vi "Send Close Event.vi"(8 "error in (no error)":errorcluster, 11 "QMenu Class in":refnum<class "QMenu Class.lvclass">) -> (0 "error out":errorcluster, 2 "Confirm":bool, 3 "QMenu Class out":refnum<class "QMenu Class.lvclass">)   [LabVIEW 2020, in "QTab.lvlib" / "QMenu Class.lvclass"]
uses:
  QMenu Class.lvclass
  QMenu Class.lvclass/QMenu Class.ctl
  Close Event Data.ctl
  Read Close Timeout.vi
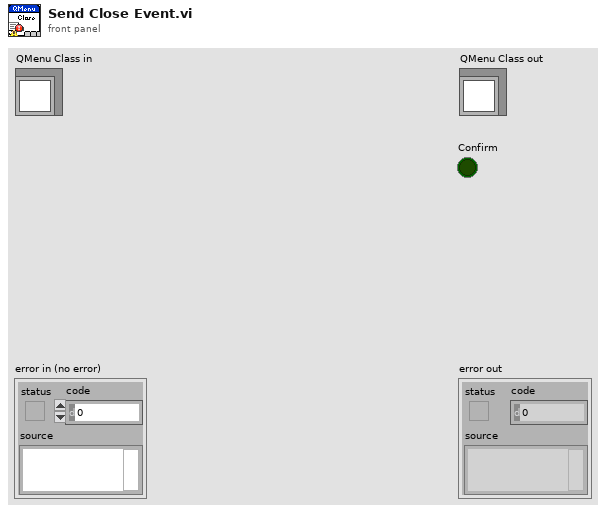
[diagram p1: front panel]
types:
  T1 = typedef "QTab.lvlib/QMenu Class.lvclass/Close Event Data.ctl" = cluster{"Index":i32, "Label":string, "Confirm Notifier":refnum<notifier>}
  T2 = typedef "QTab.lvlib/QMenu Class.lvclass/Button Attribute.ctl" = cluster{"Label":string, "Button Text":string, "Closable":bool, "Draggable":bool}
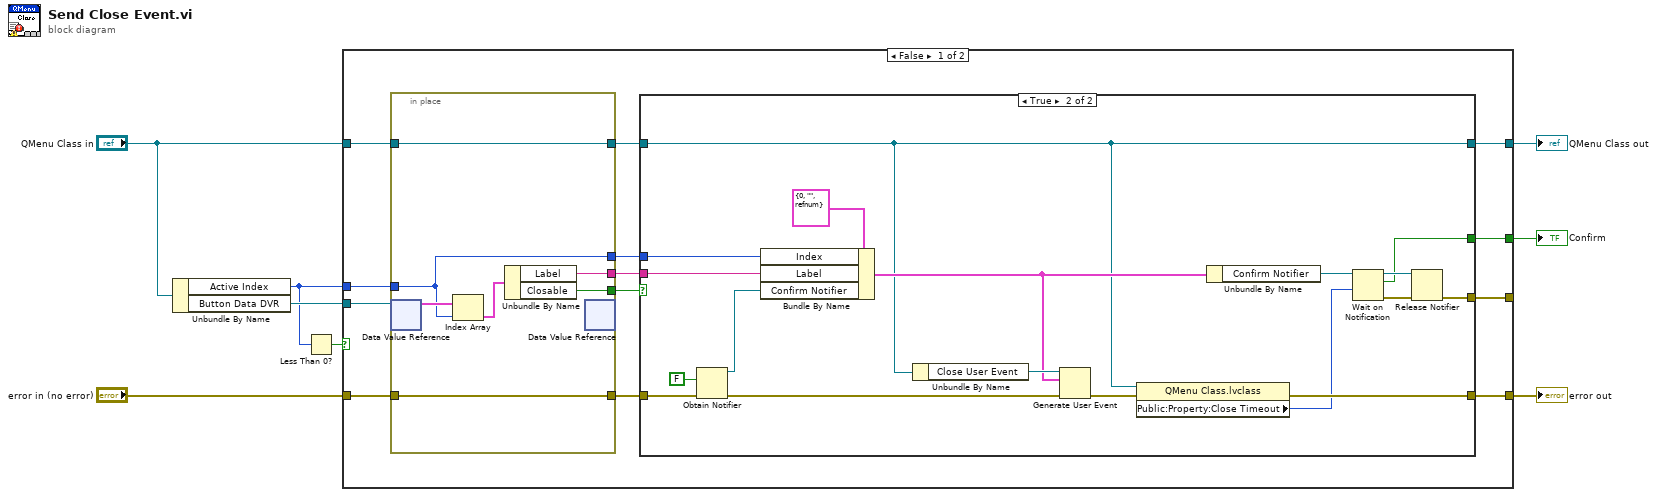
[diagram p0: block diagram]
diagram:
  n1 = Unbundle By Name("QMenu Class in") -> ("Active Index"=w3:i32, "Button Data DVR"=w7:refnum<data-value>)
  n2 = Less Than 0?(x=w3) -> (x < 0?=w2:bool)
  n3 = case shown="False" w2 {
    tunnel: [w12 w49] -> w8
    tunnel: w7 -> [w21 _]
    tunnel: "error in (no error)" -> [w20 w49]
    tunnel: "QMenu Class in" -> [w19 w50]
    tunnel: [w9 w50] -> w4
    tunnel: w3 -> [w17 _]
    tunnel: [w13 _] -> _
    tunnel: [w11 _] -> w1
    frame False {
      n4 = in-place {
        in-place-border: w17 -> [w44]
        in-place-border: w20 -> [w45]
        in-place-border: w19 -> [w48]
        in-place-border: [w48] -> w18
        in-place-border: [w45] -> w16
        in-place-border: [w44] -> w15
        in-place-border: [w43] -> w14
        in-place-border: [w42] -> w10
        n5 = in-place-dvr #1(w21) -> (w47:T2[])  [unwired: 1 out]
        n6 = Index Array(array=w47, index=w44) -> (element=w46:T2)
        n7 = Unbundle By Name(w46) -> ("Label"=w43:string, "Closable"=w42:bool)
        n8 = in-place-dvr #1() -> ()  [unwired: 1 in, 2 out]
      }
      n9 = case shown="True" w10 {
        tunnel: w18 -> [w22 w26]
        tunnel: w16 -> [w23 w40]
        tunnel: w15 -> [_ w36]
        tunnel: w14 -> [_ w35]
        tunnel: [_ w29] -> w13
        tunnel: [w23 w25] -> w12
        tunnel: [_ w28] -> w11
        tunnel: [w22 w26] -> w9
        frame False {
        }
        frame True {
          n10 = Obtain Notifier(notification data type=FALSE, error in (no error)=w40) -> (notifier out=w37:refnum<notifier>, error out=w34:errorcluster)  [unwired: 2 in, 1 out]
          n11 = Bundle By Name(cluster=T1 {"Index"=0, "Label"="", "Confirm Notifier"=refnum} ("Close Event Data"), "Index"=w36, "Label"=w35, "Confirm Notifier"=w37) -> (w33:T1)
          n12 = Unbundle By Name(w26) -> ("Close User Event"=w41:refnum<user-event>)
          n13 = Generate User Event(user event=w41, event data cluster=w33, error in=w34) -> (error out=w27:errorcluster)  [unwired: 1 in, 1 out]
          n14 = property class="QMenu Class.lvclass"(reference=w26, error in=w27) -> (error out=w25:errorcluster, "Public:Property:Close Timeout"=w24:i32)  [unwired: 1 out]
          n15 = Unbundle By Name(w33) -> ("Confirm Notifier"=w32:refnum<notifier>)
          n16 = Wait on Notification(notifier=w32, timeout in ms (-1)=w24) -> (notifier out=w31:refnum<notifier>, notification=w28:bool, error out=w30:errorcluster)  [unwired: 2 in, 1 out]
          n17 = Release Notifier(notifier=w31, error in (no error)=w30) -> (error out=w29:errorcluster)  [unwired: 1 in, 2 out]
        }
      }
    }
    frame True {
    }
  }
  "error out" <- w8
  "QMenu Class out" <- w4
  "Confirm" <- w1
